vi "aft_Check Memory Existence.vi"(8 "error in (no error)":errorcluster, 10 "name":string=" Coefficients", 11 "target ref":refnum<vi>) -> (0 "error out":errorcluster, 1 "exist?":bool, 2 "msg":string=" Coefficients", 3 "memory ref":refnum<vi>)   [LabVIEW 2017, in "NI_AdaptiveFilter.lvlib"]
uses:
  <vilib>/addons/Adaptive Filters/NI_AdaptiveFilter.lvlib
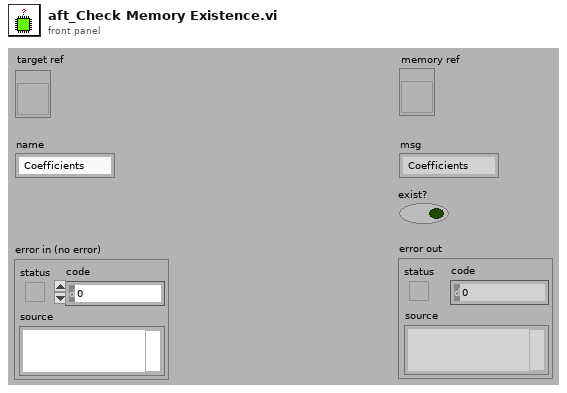
[diagram p1: front panel]
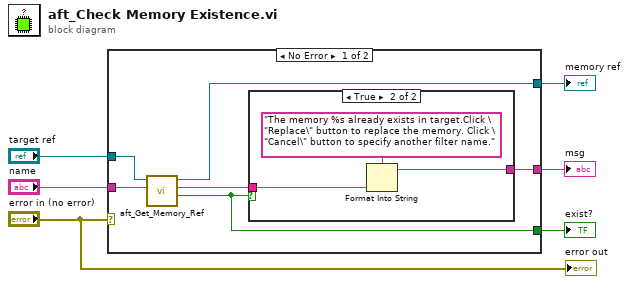
[diagram p0: block diagram]
diagram:
  n1 = case shown="No Error" "error in (no error)" {
    tunnel: "target ref" -> [w12 _]
    tunnel: "name" -> [w9 _]
    tunnel: [w11 _] -> w4
    tunnel: [w10 _] -> w3
    tunnel: [w8 _] -> w1
    frame No Error {
      n2 = call <vilib>:"aft_Get_Memory_Ref.vi"("memory name"=w9, "target ref"=w12) -> ("exist?"=w8:bool, "memory name out"=w7:string, "memory ref"=w11:refnum<vi>)  [unwired: 7 in]
      n3 = case shown="True" w8 {
        tunnel: w7 -> [_ w14]
        tunnel: [_ w13] -> w10
        frame False {
        }
        frame True {
          n4 = Format Into String(format string="The memory %s already exists in target.Click \"Replace\" button to replace the memory. Click \"Cancel\" button to specify another filter name.", w14) -> (resulting string=w13:string)  [unwired: 2 in, 1 out]
        }
      }
    }
    frame Error {
    }
  }
  "msg" <- w3
  "memory ref" <- w4
  "exist?" <- w1
  "error out" <- "error in (no error)"
